vi "Define_111_Points_In_11_Case-1.vi"(4 "error IN":errorcluster, 6 "[IN] Subtracks":T2(array[cluster]), 7 "[IN] Still connected\ntracks in group":T1) -> (0 "error OUT":errorcluster, 2 "[OUT] Indicies of subtracks \nwith \"111\" points in \"11\" case":i32[](array[numeric]))   [LabVIEW 2013]
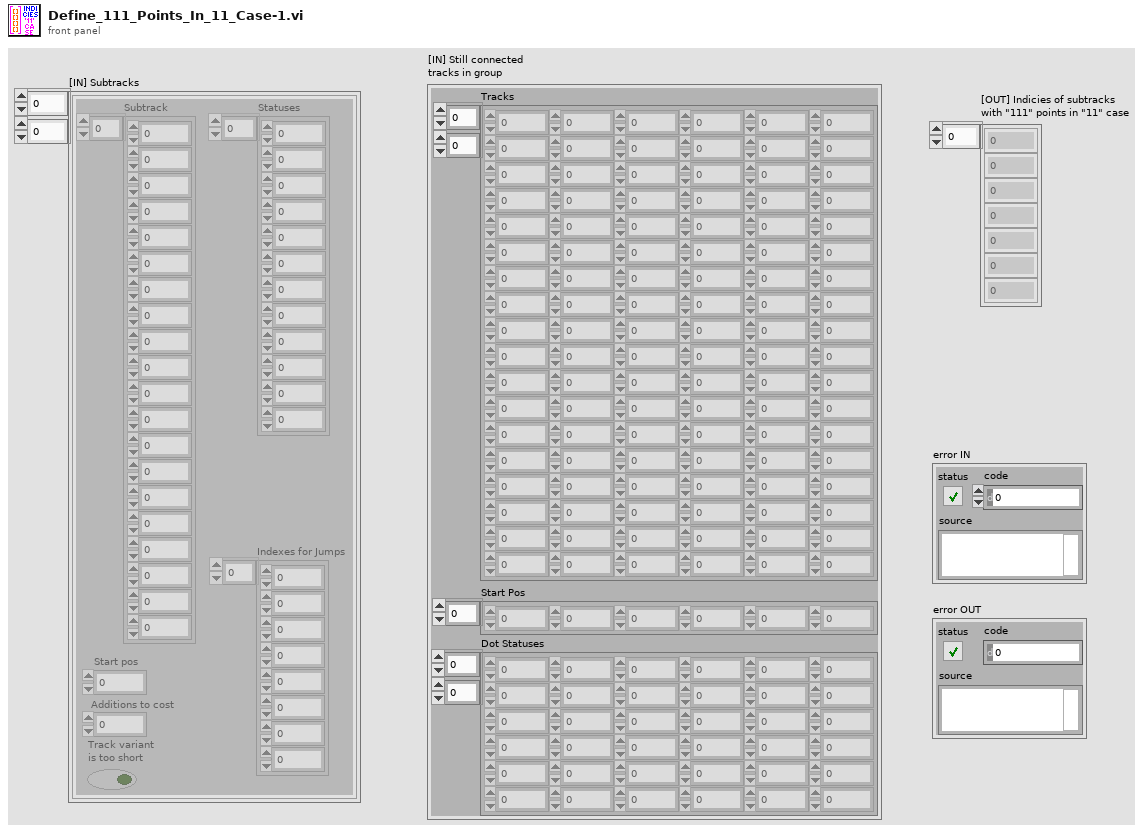
[diagram p1: front panel]
types:
  T1 = cluster{"Tracks":dbl[][], "Start Pos":i32[], "Dot Statuses":i16[][]}
  T2 = cluster{"Subtrack":dbl[], "Statuses":i16[], "Start pos":i32, "Additions to cost":i32, "Track variant \nis too short":bool, "Indexes for Jumps":i32[]}[][]
  T3 = cluster{"Subtrack":dbl[], "Statuses":i16[], "Start pos":i32, "Additions to cost":i32, "Track variant \nis too short":bool, "Indexes for Jumps":i32[]}[]
  T4 = cluster{"Subtrack":dbl[], "Statuses":i16[], "Start pos":i32, "Additions to cost":i32, "Track variant \nis too short":bool, "Indexes for Jumps":i32[]}
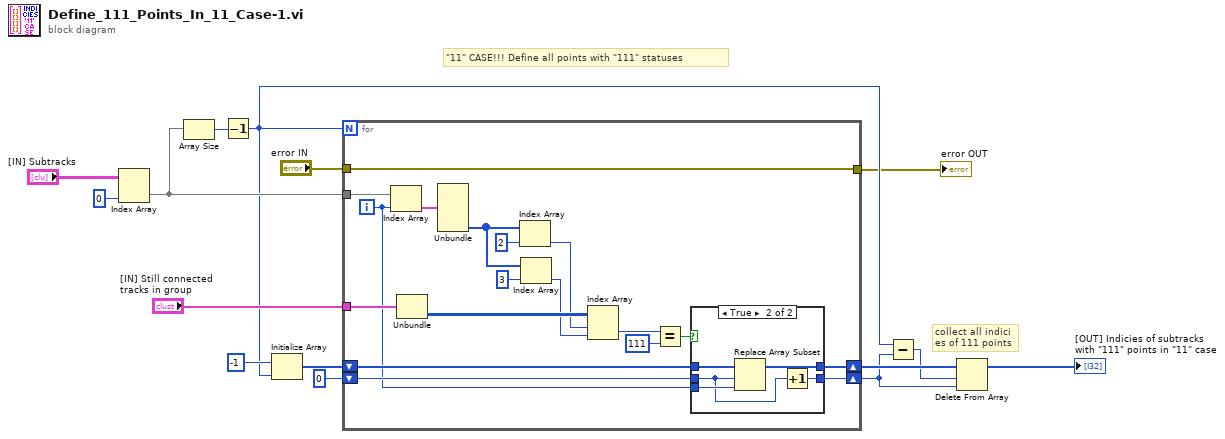
[diagram p0: block diagram]
diagram:
  # "collect all indici\nes of 111 points"
  # "\"11\" CASE!!! Define all points with \"111\" statuses"
  n1 = Index Array(array="[IN] Subtracks", index (col)=0 ("disabled index (col)")) -> (element=w11:T3)  [unwired: 1 in]
  n2 = Array Size(array=w11) -> (size(s)=w12:i32)
  n3 = Decrement(x=w12) -> (x-1=w6:i32)
  n4 = Initialize Array(-1, w6) -> (w9:i32[])
  n5 = for {
    N: w6 -> [_]
    tunnel: w11 -> [w33]
    shift-right: [w18] -> w7
    shift-left: w9 -> [w21]
    shift-right: [w17] -> w5
    shift-left: 0 -> [w20]
    tunnel: "[IN] Still connected\ntracks in group" -> [w28]
    tunnel: "error IN" -> [w16]
    tunnel: [w16] -> w2
    i -> [w19]
    n6 = Index Array(array=w33, index=w19) -> (element=w32:T4)
    n7 = Unbundle(w28) -> ("Dot Statuses"=w27:i16[][])  [unwired: 2 out]
    n8 = Unbundle(w32) -> ("Indexes for Jumps"=w29:i32[])  [unwired: 5 out]
    n9 = Index Array(array=w29, index=2) -> (element=w25:i32)
    n10 = Index Array(array=w29, index=3) -> (element=w26:i32)
    n11 = Index Array(array=w27, index (row)=w25, index (col)=w26) -> (element=w24:i16)
    n12 = Equal?(x=w24, y=i16 111) -> (x = y?=w22:bool)
    n13 = case shown="True" w22 {
      tunnel: w21 -> [w35 w40]
      tunnel: w20 -> [w34 w37]
      tunnel: w19 -> [_ w39]
      tunnel: [w35 w38] -> w18
      tunnel: [w34 w36] -> w17
      frame False {
      }
      frame True {
        n14 = Replace Array Subset(array=w40, new element=w39, index=w37) -> (w38:i32[])
        n15 = Increment(x=w37) -> (x+1=w36:i32)
      }
    }
  }
  "error OUT" <- w2
  n16 = Subtract(x=w6, y=w5) -> (x-y=w4:i32)
  n17 = Delete From Array(array=w7, length=w4, index=w5) -> (array with subset deleted=→"[OUT] Indicies of subtracks \nwith \"111\" points in \"11\" case":i32[])  [unwired: 1 out]
